vi "o3 Serial Packet Write.vi"(0 "VISA resource name In":refnum<visa-resource-name>, 7 "Data in":string, 11 "error in (no error)":errorcluster) -> (4 "VISA resource name Out":refnum<visa-resource-name>, 15 "error out":errorcluster)   [LabVIEW 2014]
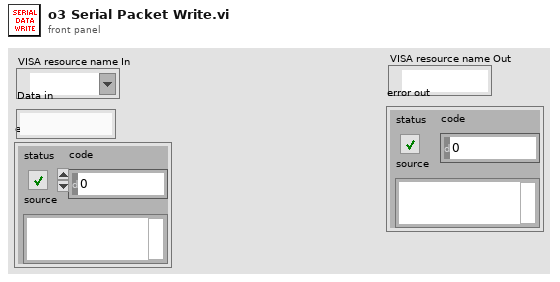
[diagram p1: front panel]
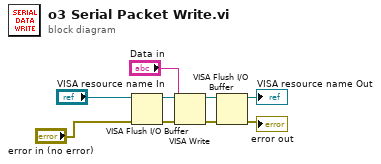
[diagram p0: block diagram]
diagram:
  n1 = VISA Flush I/O Buffer(VISA resource name="VISA resource name In", error in (no error)="error in (no error)") -> (VISA resource name out=w7:refnum<visa-resource-name>, error out=w6:errorcluster)  [unwired: 1 in]
  n2 = VISA Write(VISA resource name=w7, write buffer="Data in", error in (no error)=w6) -> (VISA resource name out=w8:refnum<visa-resource-name>, error out=w9:errorcluster)  [unwired: 1 out]
  n3 = VISA Flush I/O Buffer(VISA resource name=w8, error in (no error)=w9) -> (VISA resource name out=→"VISA resource name Out":refnum<visa-resource-name>, error out=→"error out":errorcluster)  [unwired: 1 in]
